vi "shift registers.vi"() -> ()   [LabVIEW 2020]
panel:
  out "Numeric 5":dbl
  out "Numeric 4":dbl
  out "Numeric 3":dbl
  out "Numeric 2":dbl
  in  "Numeric":dbl
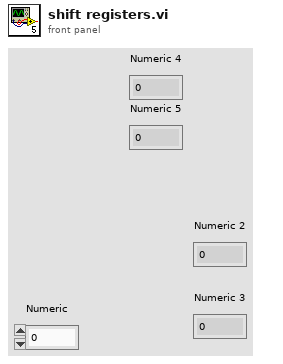
[diagram p1: front panel]
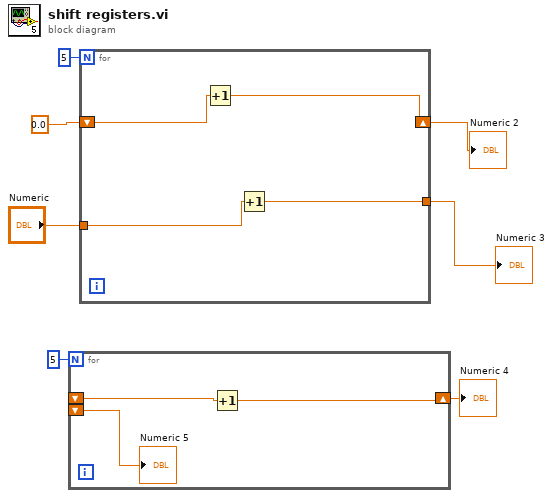
[diagram p0: block diagram]
diagram:
  n1 = for {
    N: 5 -> [_]
    shift-right: [w9] -> w2
    shift-left: _ -> [w10]
    shift-left: _ -> [w8]
    n2 = Increment(x=w10) -> (x+1=w9:dbl)
    "Numeric 5" <- w8
  }
  "Numeric 4" <- w2
  n3 = for {
    N: 5 -> [_]
    shift-right: [w13] -> w5
    shift-left: 0.0 -> [w14]
    tunnel: "Numeric" -> [w12]
    tunnel: [w11] -> w4
    n4 = Increment(x=w14) -> (x+1=w13:dbl)
    n5 = Increment(x=w12) -> (x+1=w11:dbl)
  }
  "Numeric 2" <- w5
  "Numeric 3" <- w4
